vi "SetUpQuiz.vi"(8 "Error In":errorcluster, 9 "Problem Offset (0)":i32, 10 "Quiz Set Up info":T1[](array[typedef]), 11 "? Ref Array":refnum<vi>[](array[refnum])) -> (0 "Error Out":errorcluster, 2 "Quiz Set Up Out":T1[](array[typedef]))   [LabVIEW 2012]
uses:
  Controls/StoredQuizAnswer.ctl
  Controls/Problem Type enum.ctl
  Controls/Solution Type enum.ctl
  Controls/Quiz Set Up.ctl
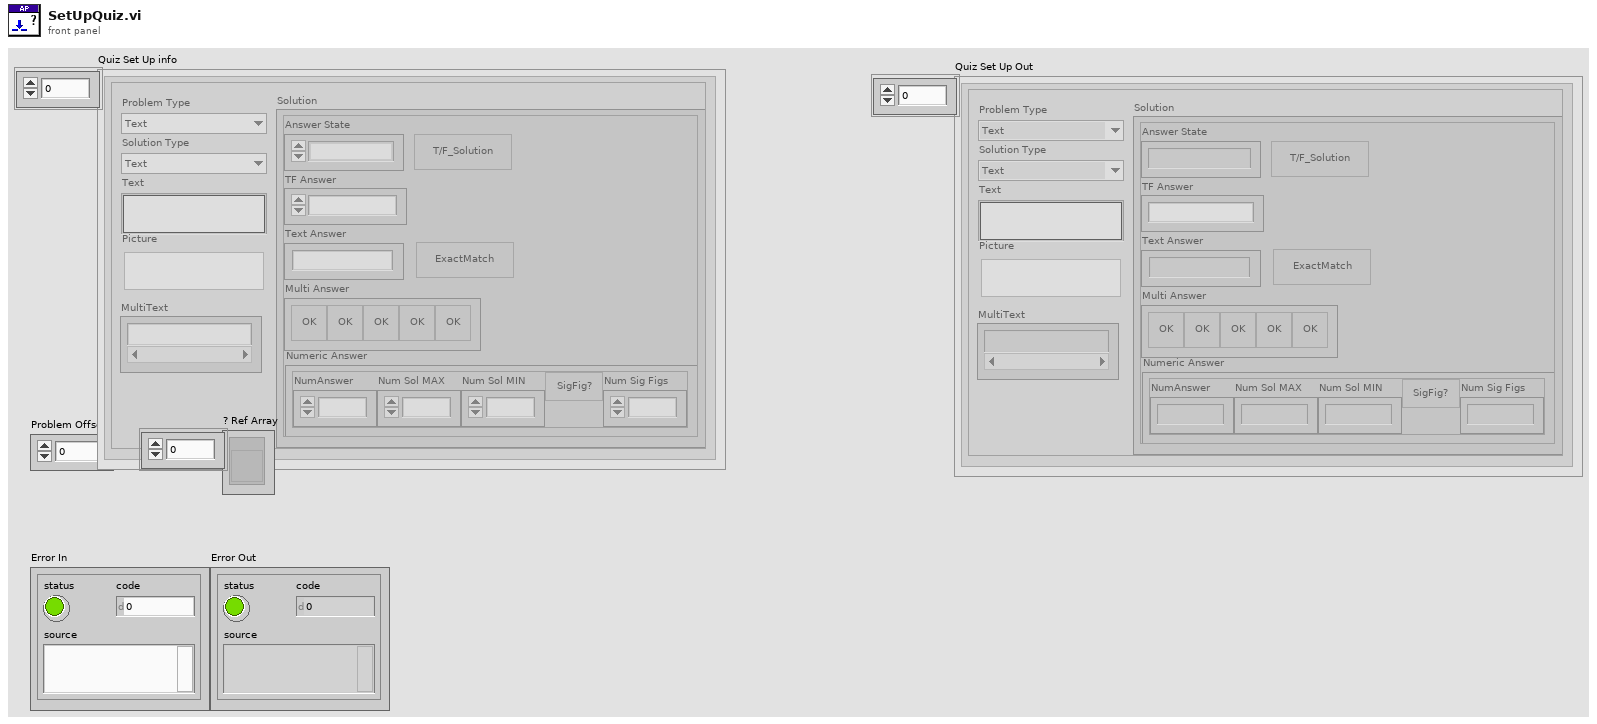
[diagram p1: front panel]
types:
  T1 = typedef "Quiz Set Up.ctl" = cluster{"Text":string, "Problem Type":T2, "Solution Type":T3, "Picture":picture, "MultiText":string[], "Solution":cluster{"Answer State":enum16{"Unanswered", "Correct", "Incorrect"}, "TF Answer":enum32{"No Selection", "True", "False"}, "Text Answer":string, "Multi Answer":bool[], "ExactMatch":bool, "Numeric Answer":cluster{"NumAnswer":dbl, "Num Sol MAX":dbl, "Num Sol MIN":dbl, "SigFig?":bool, "Num Sig Figs":i32}, "T/F_Solution":bool}}
  T2 = typedef "Problem Type enum.ctl" = enum16{"Text", "Image", "Text&Image"}
  T3 = typedef "Solution Type enum.ctl" = enum16{"Numeric", "Text", "SelectMultiple", "SelectOne", "True/False", "ShortAnswer"}
  T4 = typedef "StoredQuizAnswer.ctl" = cluster{"ShortAnswer":string, "TrueFalseAnswer":enum32{"No Selection", "True", "False"}, "RadioAnswer":enum32{"No Selection", "Radio Selection A", "Radio Selection B", "Radio Selection C", "Radio Selection D", "Radio Selection E"}, "MultiAnswer":cluster{"MultiAnswer":bool[], "MultiText":string[]}, "StringAnswer":string, "NumAnswer":dbl}
  T5 = enum8{"Enabled", "Disabled", "Disabled and Grayed Out"}
  T6 = cluster{"NumAnswer":dbl, "StringAnswer":string, "MultiAnswer":cluster{"MultiAnswer":bool[], "MultiText":string[]}, "RadioAnswer":enum32{"No Selection", "Radio Selection A", "Radio Selection B", "Radio Selection C", "Radio Selection D", "Radio Selection E"}, "TrueFalseAnswer":enum32{"No Selection", "True", "False"}, "ShortAnswer":string}
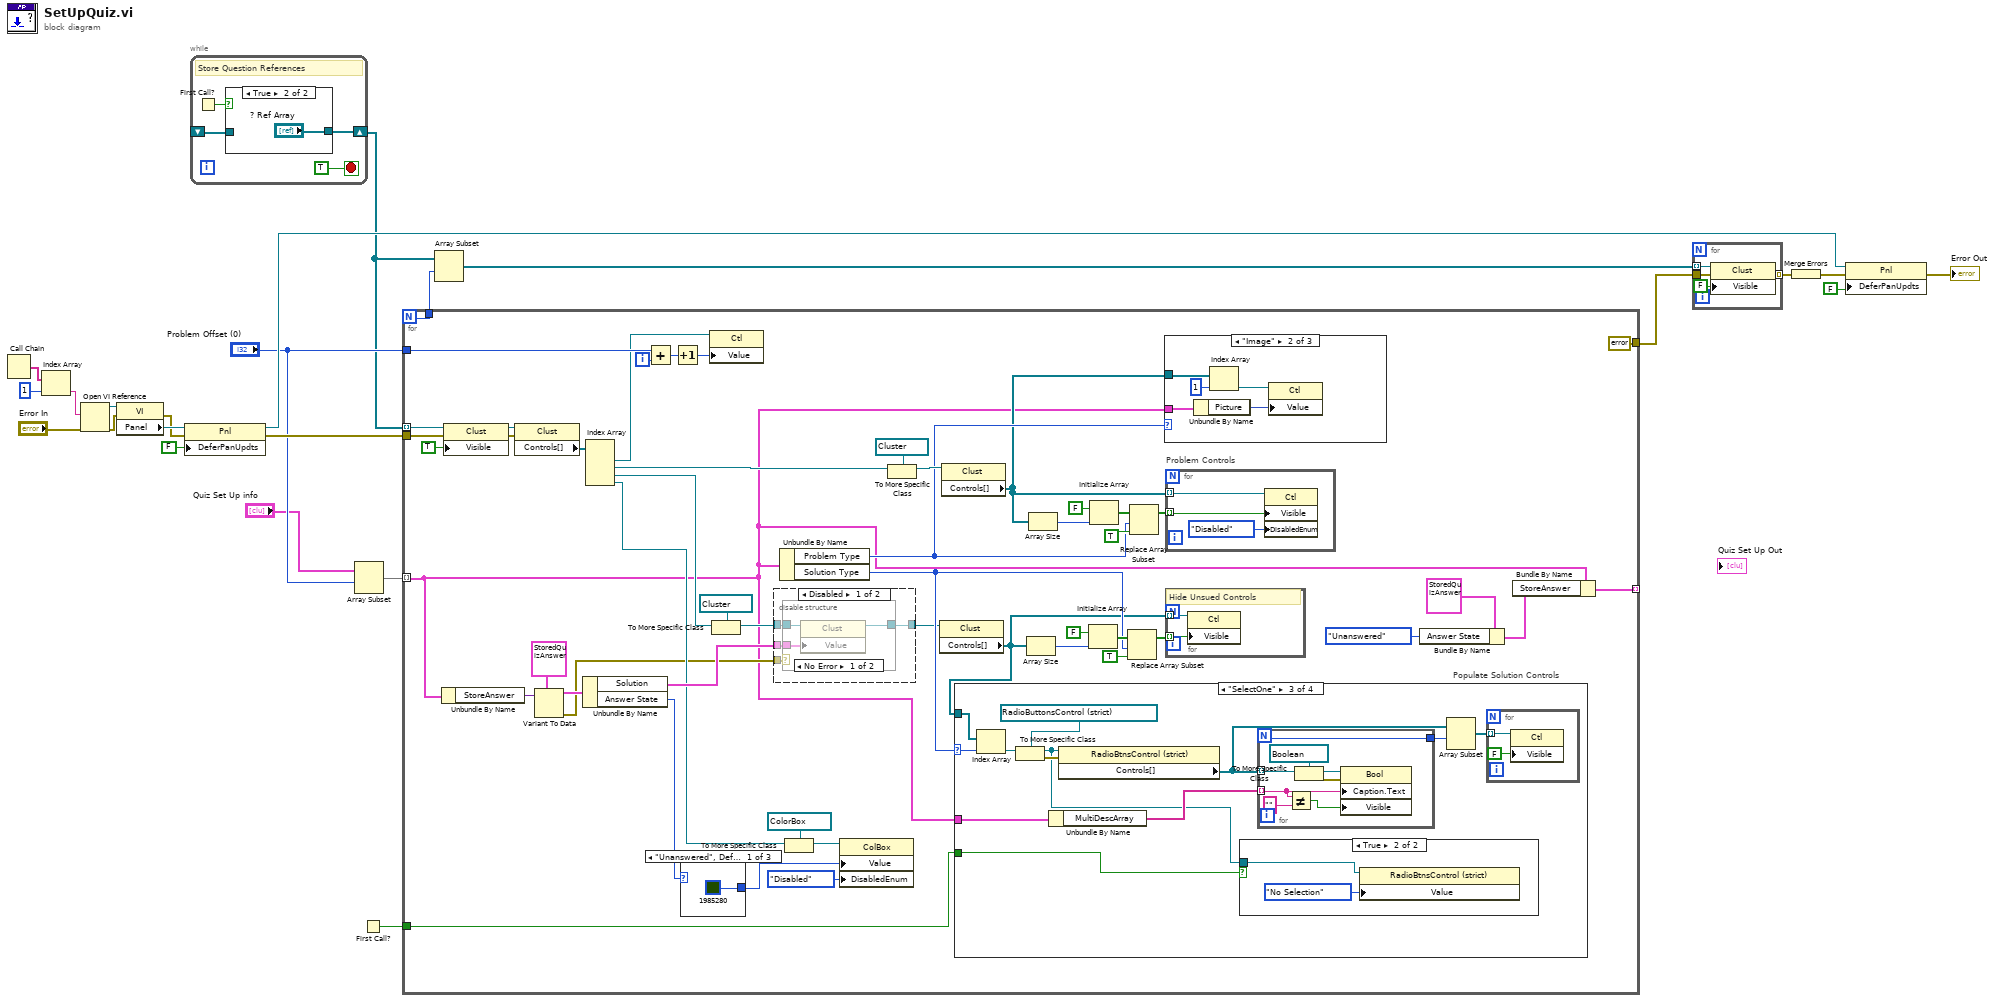
[diagram p0: block diagram]
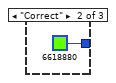
[diagram p5: hidden frame]
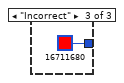
[diagram p6: hidden frame]
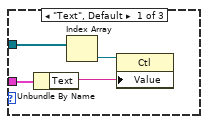
[diagram p7: hidden frame]
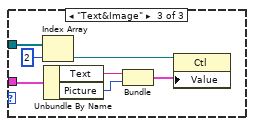
[diagram p8: hidden frame]
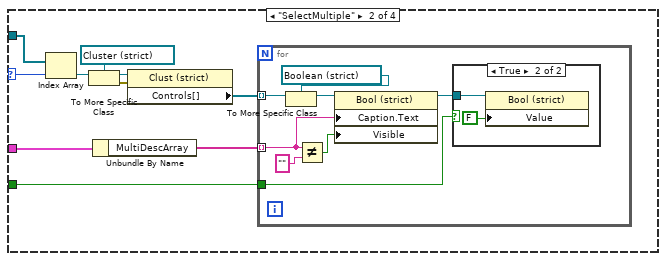
[diagram p10: hidden frame]
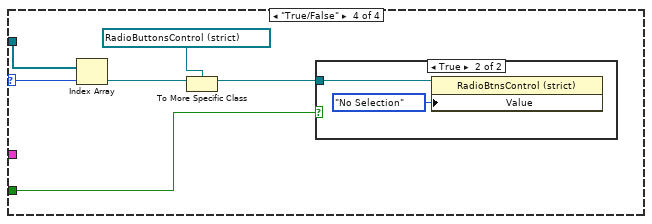
[diagram p13: hidden frame]
diagram:
  n1 = Call Chain() -> (call chain=w8:string[])
  n2 = Index Array(array=w8, index=1) -> (element=w6:string)
  n3 = Open VI Reference(vi path=w6, error in (no error)="Error In") -> (vi reference=w16:refnum<vi>, error out=w13:errorcluster)  [unwired: 4 in]
  n4 = property class="VI"(reference=w16, error in=w13) -> (error out=w14:errorcluster, "Panel"=w21:refnum<vi>)  [unwired: 1 out]
  n5 = property class="Pnl"(reference=w21, error in=w14, "DeferPanUpdts"=FALSE ("Defer Panel Updates")) -> (reference out=w18:refnum<vi>, error out=w19:errorcluster)
  n6 = while {
    shift-right: [w27] -> w2
    shift-left: _ -> [w26]
    stop <- TRUE stop-if-true
    # "Store Question References"
    n7 = First Call?() -> (First Call?: T/F=w25:bool)
    n8 = case shown="True" w25 {
      tunnel: [w28 "? Ref Array"] -> w27
      tunnel: w26 -> [w28 _]
      frame False {
      }
      frame True {
      }
    }
  }
  n9 = Array Subset(array="Quiz Set Up info", index="Problem Offset (0)") -> (w15:T1[])  [unwired: 1 in]
  n10 = First Call?() -> (First Call?: T/F=w9:bool)
  n11 = for {
    N -> [w61]
    tunnel: w2 -> [w59] mode=indexing
    tunnel: w15 -> [w34] mode=indexing
    tunnel: [w61] -> w23
    tunnel: w19 -> [w52]
    tunnel: [errorcluster {"status"=FALSE, "code"=0, "source"=""} ("error in (no error)")] -> w12
    tunnel: "Problem Offset (0)" -> [w53]
    tunnel: w9 -> [w44]
    tunnel: [w30] -> _ mode=indexing
    i -> [w62]
    n12 = Unbundle By Name(w34) -> ("StoreAnswer"=w57:variant)
    n13 = property on="Property Node" class="Clust"(reference=w59, error in=w52, "Visible"=TRUE) -> (reference out=w43:refnum<vi>, error out=w42:errorcluster)
    n14 = property on="Property Node" class="Clust"(reference=w43, error in=w42) -> ("Controls[]"=w76:refnum<vi>[])  [unwired: 2 out]
    n15 = Variant To Data(type=T4 {"ShortAnswer"="", "TrueFalseAnswer"=enum."No Selection", "RadioAnswer"=enum."No Selection", "MultiAnswer"={"MultiAnswer"=[], "MultiText"=[]}, "StringAnswer"="", "NumAnswer"=0.0} ("output cluster"), Variant=w57) -> (data=w51:T4, error out=w35:errorcluster)  [unwired: 1 in]
    n16 = Unbundle By Name(w51) -> ("Solution"=w50:T6, "Answer State"=w38:enum16{"Unanswered", "Correct", "Incorrect"})
    n17 = Index Array(array=w76) -> (element #1=w41:refnum<vi>, element #2=w40:refnum<vi>, element #3=w39:refnum<vi>, element #4=w36:refnum<vi>)  [unwired: 4 in]
    n18 = Add(x=w53, y=w62) -> (x+y=w54:i32)
    n19 = Increment(x=w54) -> (x+1=w63:i32)
    n20 = case shown="\"Unanswered\", Default" w38 {
      tunnel: [u32 1985280 u32 6618880 u32 16711680] -> w37
      frame "Unanswered", Default {
      }
      frame "Correct" {
      }
      frame "Incorrect" {
      }
    }
    n21 = property on="Property Node" class="Ctl"(reference=w41, "Value"=w63) -> ()  [unwired: 1 in, 2 out]
    n22 = To More Specific Class(target class=refnum<vi> refnum ("Problem Type"), reference=w39) -> (specific class reference=w56:refnum<vi>)  [unwired: 1 in, 1 out]
    n23 = disable-structure shown="Disabled" {
      disable-tunnel: w56 -> [w84 w89]
      disable-tunnel: [w83 w89] -> w55
      disable-tunnel: w50 -> [w82 _]
      disable-tunnel: w35 -> [w81 _]
      frame Disabled {
        n24 = case shown="No Error" w81 {
          tunnel: w84 -> [w87 w88]
          tunnel: [w86 w88] -> w83
          tunnel: w82 -> [w85 _]
          frame No Error {
            n25 = property class="Clust"(reference=w87, "Value"=w85) -> (reference out=w86:refnum<vi>)  [unwired: 1 in, 1 out]
          }
          frame Error {
          }
        }
      }
      frame Enabled {
      }
    }
    n26 = Unbundle By Name(w34) -> ("Problem Type"=w69:T2, "Solution Type"=w70:T3)
    n27 = To More Specific Class(target class=refnum<vi> refnum ("Problem Type"), reference=w36) -> (specific class reference=w48:refnum<vi>)  [unwired: 1 in, 1 out]
    n28 = property class="ColBox"(reference=w48, "Value"=w37, "DisabledEnum"=T5."Disabled" ("Disabled")) -> ()  [unwired: 1 in, 2 out]
    n29 = To More Specific Class(target class=refnum<vi> refnum ("Problem Type"), reference=w40) -> (specific class reference=w80:refnum<vi>)  [unwired: 1 in, 1 out]
    n30 = property on="Property Node" class="Clust"(reference=w55) -> ("Controls[]"=w46:refnum<vi>[])  [unwired: 1 in, 2 out]
    n31 = property on="Property Node" class="Clust"(reference=w80) -> ("Controls[]"=w67:refnum<vi>[])  [unwired: 1 in, 2 out]
    n32 = case "Populate Solution Controls" shown="\"SelectOne\"" w70 {
      selector: w70 -> [_ w116 w133 w157]
      tunnel: w34 -> [_ w118 w137 _]
      tunnel: w46 -> [_ w117 w134 w158]
      tunnel: w44 -> [_ w110 w132 w154]
      frame "Numeric", Default {
      }
      frame "SelectMultiple" {
        n33 = Index Array(array=w117, index=w116) -> (element=w115:refnum<vi>)
        n34 = To More Specific Class(target class=refnum<vi> refnum ("Multi"), reference=w115) -> (specific class reference=w114:refnum<vi>, error out=w113:errorcluster)  [unwired: 1 in]
        n35 = Unbundle By Name(w118) -> ("MultiDescArray"=w111:string[])
        n36 = property on="Property Node" class="Clust (strict)"(reference=w114, error in=w113) -> ("Controls[]"=w112:refnum<vi>[])  [unwired: 2 out]
        n37 = for {
          tunnel: w112 -> [w126] mode=indexing
          tunnel: w111 -> [w124] mode=indexing
          tunnel: w110 -> [w121]
          n38 = To More Specific Class(target class=refnum<vi> refnum ("A"), reference=w126) -> (specific class reference=w125:refnum<vi>)  [unwired: 1 in, 1 out]
          n39 = Not Equal?(x=w124, y="") -> (x != y?=w122:bool)
          n40 = property on="Property Node" class="Bool (strict)"(reference=w125, "Caption.Text"=w124, "Visible"=w122) -> (reference out=w120:refnum<vi>)  [unwired: 1 in, 1 out]
          n41 = case shown="True" w121 {
            tunnel: w120 -> [_ w128]
            frame False {
            }
            frame True {
              n42 = property on="Property Node" class="Bool (strict)"(reference=w128, "Value"=FALSE) -> ()  [unwired: 1 in, 2 out]
            }
          }
        }
      }
      frame "SelectOne" {
        n43 = Index Array(array=w134, index=w133) -> (element=w131:refnum<vi>)
        n44 = To More Specific Class(target class=refnum<vi> refnum ("Radio"), reference=w131) -> (specific class reference=w130:refnum<vi>, error out=w138:errorcluster)  [unwired: 1 in]
        n45 = Unbundle By Name(w137) -> ("MultiDescArray"=w136:string[])
        n46 = property on="Property Node" class="RadioBtnsControl (strict)"(reference=w130, error in=w138) -> ("Controls[]"=w139:refnum<vi>[])  [unwired: 2 out]
        n47 = case shown="True" w132 {
          tunnel: w130 -> [_ w142]
          frame False {
          }
          frame True {
            n48 = property on="Property Node" class="RadioBtnsControl (strict)"(reference=w142, "Value"=enum32{"No Selection", "A", "B", "C", "D", "E"}."No Selection") -> ()  [unwired: 1 in, 2 out]
          }
        }
        n49 = for {
          N -> [w148]
          tunnel: w136 -> [w147] mode=indexing
          tunnel: w139 -> [w152] mode=indexing
          tunnel: [w148] -> w140
          n50 = Not Equal?(x=w147, y="") -> (x != y?=w145:bool)
          n51 = To More Specific Class(target class=refnum<vi> refnum ("Problem Type"), reference=w152) -> (specific class reference=w151:refnum<vi>, error out=w149:errorcluster)  [unwired: 1 in]
          n52 = property on="Property Node" class="Bool"(reference=w151, error in=w149, "Caption.Text"=w147, "Visible"=w145) -> ()  [unwired: 2 out]
        }
        n53 = Array Subset(array=w139, index=w140) -> (w135:refnum<vi>[])  [unwired: 1 in]
        n54 = for {
          tunnel: w135 -> [w143] mode=indexing
          n55 = property on="Property Node" class="Ctl"(reference=w143, "Visible"=FALSE) -> ()  [unwired: 1 in, 2 out]
        }
      }
      frame "True/False" {
        n56 = Index Array(array=w158, index=w157) -> (element=w156:refnum<vi>)
        n57 = To More Specific Class(target class=refnum<vi> refnum ("True/False"), reference=w156) -> (specific class reference=w155:refnum<vi>)  [unwired: 1 in, 1 out]
        n58 = case shown="True" w154 {
          tunnel: w155 -> [_ w160]
          frame False {
          }
          frame True {
            n59 = property on="Property Node" class="RadioBtnsControl (strict)"(reference=w160, "Value"=enum32{"No Selection", "True", "False"}."No Selection") -> ()  [unwired: 1 in, 2 out]
          }
        }
      }
    }
    n60 = Array Size(array=w46) -> (size(s)=w75:i32)
    n61 = Array Size(array=w67) -> (size(s)=w68:i32)
    n62 = Initialize Array(FALSE, w75) -> (w73:bool[])
    n63 = Initialize Array(FALSE, w68) -> (w65:bool[])
    n64 = Replace Array Subset(array=w73, new element=TRUE, index=w70) -> (w72:bool[])
    n65 = Replace Array Subset(array=w65, new element=TRUE, index=w69) -> (w77:bool[])
    n66 = case shown="\"Image\"" w69 {
      tunnel: w67 -> [w96 w100 w106]
      tunnel: w34 -> [w94 w101 w108]
      frame "Text", Default {
        n67 = Unbundle By Name(w94) -> ("Text"=w93:string)
        n68 = Index Array(array=w96) -> (element=w95:refnum<vi>)  [unwired: 1 in]
        n69 = property on="Property Node" class="Ctl"(reference=w95, "Value"=w93) -> ()  [unwired: 1 in, 2 out]
      }
      frame "Image" {
        n70 = Unbundle By Name(w101) -> ("Picture"=w97:picture)
        n71 = Index Array(array=w100, index=1) -> (element=w98:refnum<vi>)
        n72 = property on="Property Node" class="Ctl"(reference=w98, "Value"=w97) -> ()  [unwired: 1 in, 2 out]
      }
      frame "Text&Image" {
        n73 = Index Array(array=w106, index=2) -> (element=w104:refnum<vi>)
        n74 = Unbundle By Name(w108) -> ("Text"=w107:string, "Picture"=w102:picture)
        n75 = Bundle("Text"=w107, "Picture"=w102) -> (w103:cluster{"Text":string, "Picture":picture})  [unwired: 1 in]
        n76 = property on="Property Node" class="Ctl"(reference=w104, "Value"=w103) -> ()  [unwired: 1 in, 2 out]
      }
    }
    n77 = for "Problem Controls" {
      tunnel: w67 -> [w165] mode=indexing
      tunnel: w77 -> [w164] mode=indexing
      n78 = property on="Property Node" class="Ctl"(reference=w165, "Visible"=w164, "DisabledEnum"=T5."Disabled" ("Disabled")) -> ()  [unwired: 1 in, 2 out]
    }
    n79 = for "Solution Controls" {
      tunnel: w46 -> [w162] mode=indexing
      tunnel: w72 -> [w161] mode=indexing
      # "Hide Unsued Controls"
      n80 = property on="Property Node" class="Ctl"(reference=w162, "Visible"=w161) -> ()  [unwired: 1 in, 2 out]
    }
    n81 = Bundle By Name(cluster=T4 {"ShortAnswer"="", "TrueFalseAnswer"=enum."No Selection", "RadioAnswer"=enum."No Selection", "MultiAnswer"={"MultiAnswer"=[], "MultiText"=[]}, "StringAnswer"="", "NumAnswer"=0.0} ("output cluster"), "Answer State"=enum16{"Unanswered", "Correct", "Incorrect"}."Unanswered") -> (w32:T4)
    n82 = Bundle By Name(cluster=w34, "StoreAnswer"=w32) -> (w30:T1)
  }
  n83 = Array Subset(array=w2, index=w23) -> (w22:refnum<vi>[])  [unwired: 1 in]
  n84 = for {
    tunnel: w22 -> [w168] mode=indexing
    tunnel: w12 -> [w167]
    tunnel: [w166] -> w11 mode=indexing
    n85 = property on="Property Node" class="Clust"(reference=w168, error in=w167, "Visible"=FALSE) -> (error out=w166:errorcluster)  [unwired: 1 out]
  }
  n86 = Merge Errors(w11) -> (w10:errorcluster)
  n87 = property class="Pnl"(reference=w18, error in=w10, "DeferPanUpdts"=FALSE ("Defer Panel Updates")) -> (error out=→"Error Out":errorcluster)  [unwired: 1 out]
